vi "controlLinearization.vi"(7 "set":bool, 8 "error in":errorcluster, 10 "LutUsageEnable":bool, 11 "connection ID in":i32) -> (0 "error out":errorcluster, 2 "LutUsageEnable out":bool, 3 "connection ID":i32)   [LabVIEW 2016]
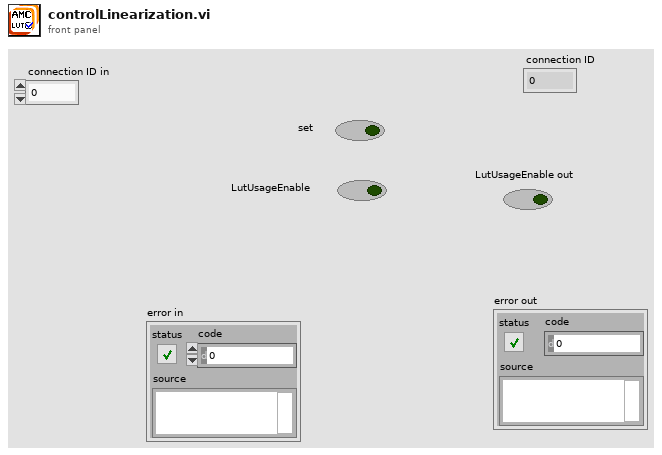
[diagram p1: front panel]
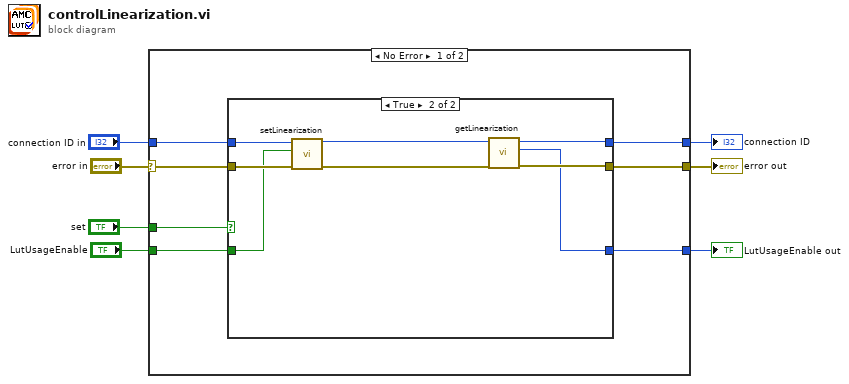
[diagram p0: block diagram]
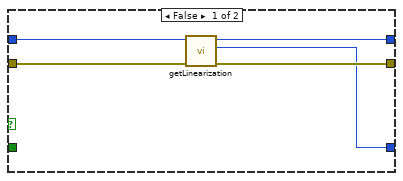
[diagram p2: hidden frame]
diagram:
  n1 = case shown="No Error" "error in" {
    selector: "error in" -> [w10 w29]
    tunnel: [w11 w30] -> w6
    tunnel: "connection ID in" -> [w12 w30]
    tunnel: [w9 w29] -> w4
    tunnel: "set" -> [w14 _]
    tunnel: "LutUsageEnable" -> [w13 w28]
    tunnel: [w8 w28] -> w1
    frame No Error {
      n2 = case shown="True" w14 {
        tunnel: w13 -> [_ w25]
        tunnel: w12 -> [w19 w27]
        tunnel: [w17 w22] -> w11
        tunnel: w10 -> [w18 w26]
        tunnel: [w16 w23] -> w9
        tunnel: [w15 w20] -> w8
        frame False {
          n3 = call "getLinearization.vi"("error in"=w18, "connection ID"=w19) -> ("error out"=w16:errorcluster, "axis_out"=w15:i32, "connection ID"=w17:i32)  [unwired: 6 in, 1 out]
        }
        frame True {
          n4 = call "setLinearization.vi"("error in"=w26, "axis"=w25, "connection ID"=w27) -> ("error out"=w24:errorcluster, "connection ID"=w21:i32)  [unwired: 6 in, 1 out]
          n5 = call "getLinearization.vi"("error in"=w24, "connection ID"=w21) -> ("error out"=w23:errorcluster, "axis_out"=w20:i32, "connection ID"=w22:i32)  [unwired: 6 in, 1 out]
        }
      }
    }
    frame Error {
    }
  }
  "connection ID" <- w6
  "error out" <- w4
  "LutUsageEnable out" <- w1
